vi "FA_MultiWriteETag.vi"(6 "Error In":errorcluster, 7 "eTag Array":string[](array[string]), 8 "ID Array":string[](array[string])) -> (0 "Error Out":errorcluster)   [LabVIEW 2013, in "FA_LocalStore.lvlib"]
doc: "Given an array of Special Type this VI writes a new eTags for each special type to the LocalStore."
uses:
  FA_LocalStore.lvlib
  <vilib>/Utility/config.llb/Write Key (String).vi
  <vilib>/Utility/config.llb/NI_LVConfig.lvlib
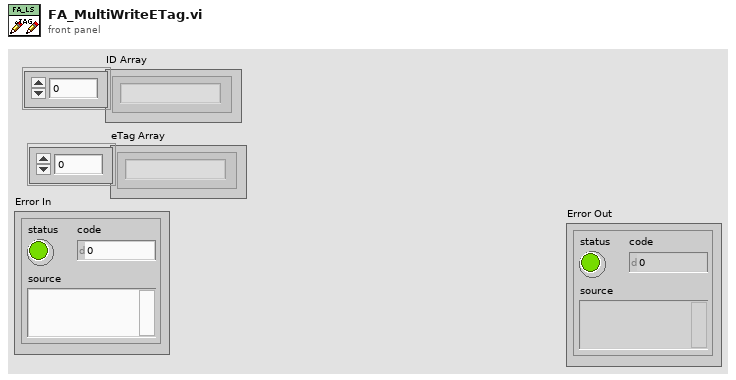
[diagram p1: front panel]
types:
  T1 = typedef "FA_LocalStore.lvlib/FA_LSRef.ctl" = cluster{"eTag INI Refnum":T2, "XML Refnum Array":refnum<file>[]}
  T2 = typedef "NI_LVConfig.lvlib/Config Data RefNum.ctl" = refnum<k1>
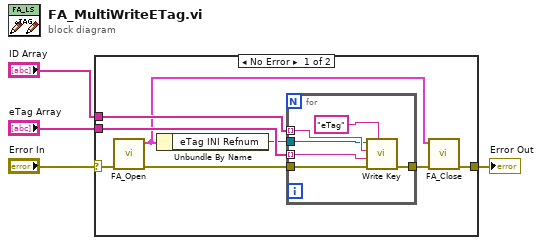
[diagram p0: block diagram]
diagram:
  n1 = case shown="No Error" "Error In" {
    selector: "Error In" -> [w8 w19]
    tunnel: [w9 w19] -> w4
    tunnel: "ID Array" -> [w11 _]
    tunnel: "eTag Array" -> [w12 _]
    frame No Error {
      n2 = call "FA_Open.vi"("Error In"=w8) -> ("Error Out"=w7:errorcluster, "FA_LS Ref"=w6:T1)  [unwired: 9 in]
      n3 = Unbundle By Name(w6) -> ("eTag INI Refnum"=w5:T2)
      n4 = for {
        tunnel: w12 -> [w17] mode=indexing
        tunnel: w11 -> [w16] mode=indexing
        tunnel: [w15] -> w10
        tunnel: w7 -> [w14]
        tunnel: w5 -> [w13]
        n5 = call-poly <vilib>:"Write Key.vi"("section"="eTag", "error in (no error)"=w14, "value"=w17, "key"=w16, "refnum"=w13) -> ("error out"=w15:errorcluster)  [unwired: 4 in, 2 out]
      }
      n6 = call "FA_Close.vi"("Error In"=w10, "FA_LS Ref"=w6) -> ("Error Out"=w9:errorcluster)  [unwired: 9 in]
    }
    frame Error {
    }
  }
  "Error Out" <- w4
